vi "play sound rt.vi"() -> ()   [LabVIEW 2026]
uses:
  <vilib>/Analysis/1siggen.llb/Ramp Pattern by Samples.vi
  68eb3da8-f18c-44af-9a6e-03eb1aa6e4d3.vi
  <vilib>/DAQmx/write.llb/DAQmx Write (Analog Wfm 1Chan NSamp).vi
  <vilib>/DAQmx/create/channels.llb/DAQmx Create Channel (AO-Voltage-Basic).vi
  <vilib>/DAQmx/configure/timing.llb/DAQmx Timing (Sample Clock).vi
  <vilib>/DAQmx/miscellaneous.llb/DAQmx Fill In Error Info.vi
  <resource>/objmgr/daqmx.rc
  <vilib>/Analysis/NI_AALBase.lvlib
panel:
  out "error out":errorcluster
  in  "stop":bool
  in  "Boolean":bool
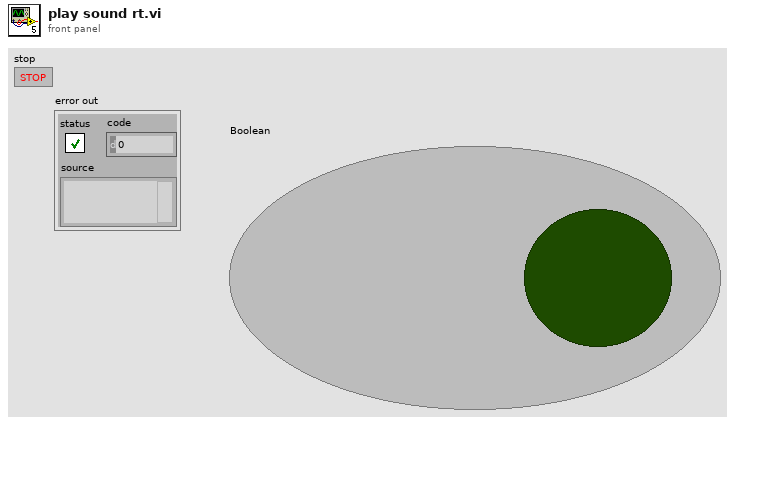
[diagram p1: front panel]
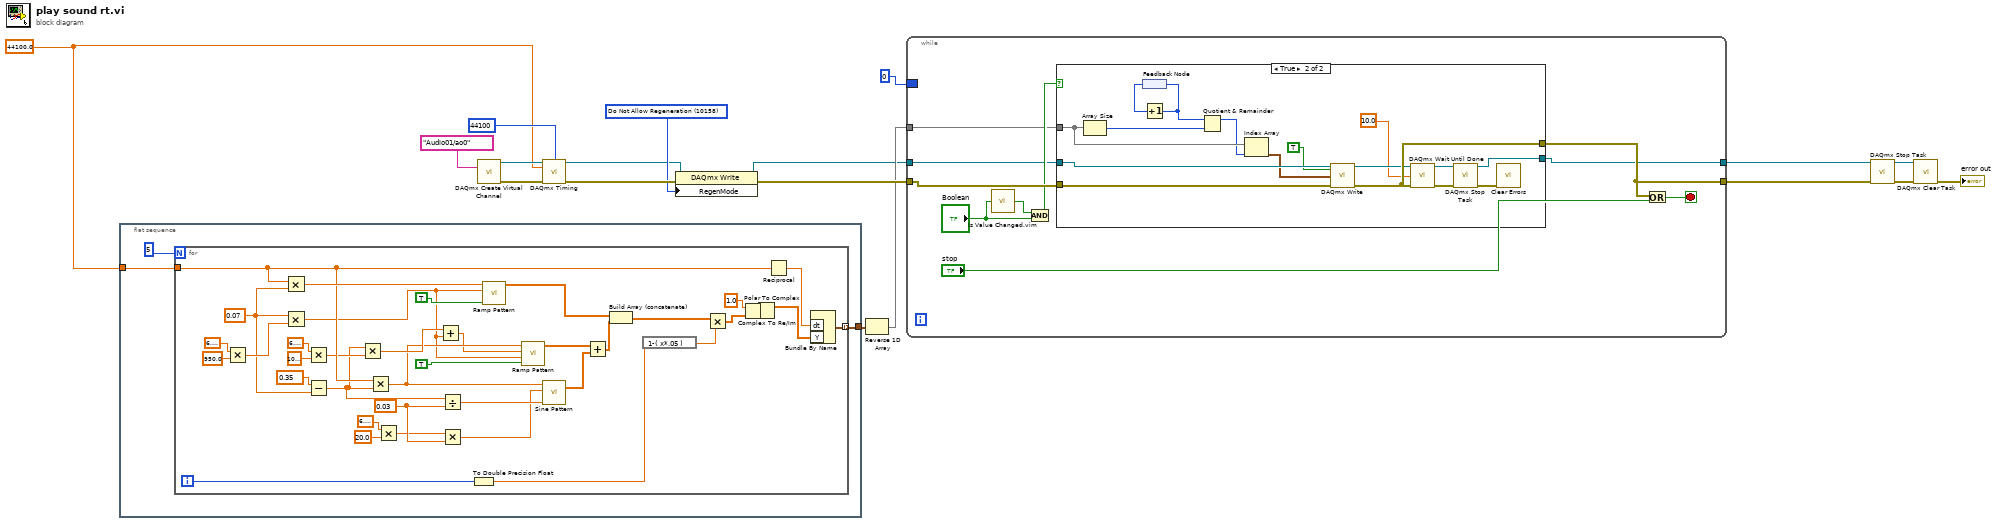
[diagram p0: block diagram]
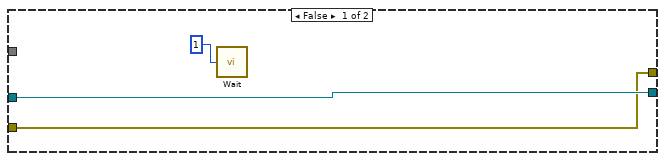
[diagram p2: hidden frame]
diagram:
  w7 = 10158 items=["Allow Regeneration"=10097, "Do Not Allow Regeneration"=10158] ("RegenMode")
  w5 = 44100.0 ("rate")
  n1 = flat-sequence {
    tunnel: [w21] -> w6
    tunnel: w5 -> [w20]
    frame #0 {
      n2 = for {
        N: 5 -> [_]
        tunnel: [w49] -> w21 mode=indexing
        tunnel: w20 -> [w45]
        i -> [w24]
        w33 = 0.03 ("y")
        w35 = 0.07 ("y")
        n3 = Multiply(x=6.283185307179586, y=950.0) -> (x*y=w55:dbl)
        n4 = Multiply(x=w45, y=w35) -> (x*y=w48:dbl)
        n5 = Multiply(x=w35, y=w55) -> (x*y=w26:dbl)
        n6 = Multiply(x=6.283185307179586, y=1000.0) -> (x*y=w41:dbl)
        n7 = Subtract(x=0.35 ("y"), y=w35) -> (x-y=w30:dbl)
        n8 = Multiply(x=w30, y=w41) -> (x*y=w47:dbl)
        n9 = Multiply(x=w45, y=w30) -> (x*y=w36:dbl)
        n10 = Multiply(x=6.283185307179586, y=20.0) -> (x*y=w32:dbl)
        n11 = Add(x=w47, y=w26) -> (x+y=w27:dbl)
        n12 = Divide(x=w30, y=w33) -> (x/y=w39:dbl)
        n13 = Multiply(x=w32, y=w33) -> (x*y=w31:dbl)
        n14 = To Double Precision Float(number=w24) -> (double precision float=w22:dbl)
        n15 = call-poly <vilib>:"Ramp Pattern.vi"("exclude end?"=TRUE, "end"=w26, "samples"=w48) -> ("Ramp Pattern"=w56:dbl[])  [unwired: 7 in, 1 out]
        n16 = call-poly <vilib>:"Ramp Pattern.vi"("exclude end?"=TRUE, "start"=w26, "end"=w27, "samples"=w36) -> ("Ramp Pattern"=w44:dbl[])  [unwired: 6 in, 1 out]
        n17 = call <vilib>:"Sine Pattern.vi"("cycles"=w39, "amplitude"=w31, "samples"=w36) -> ("Sinusoidal Pattern"=w34:dbl[])  [unwired: 1 in, 1 out]
        n18 = Add(x=w44, y=w34) -> (x+y=w28:dbl[])
        n19 = Build Array (concatenate)(w56, w28) -> (w29:dbl[])
        n20 = expression code="1-( x*.05 )"(w22) -> (w23:dbl)
        n21 = Multiply(x=w29, y=w23) -> (x*y=w25:dbl[])
        n22 = Polar To Complex(1:w25, 2:1.0 ("y")) -> (0:w52:cdb[])
        n23 = Complex To Re/Im(x + iy=w52) -> (x=w51:dbl[])  [unwired: 1 out]
        n24 = Reciprocal(x=w45) -> (1/x=w50:dbl)
        n25 = Bundle By Name("dt"=w50, "Y"=w51) -> (w49:waveform(dbl))  [unwired: 1 in]
      }
    }
  }
  n26 = call-poly <vilib>:"DAQmx Create Virtual Channel.vi"("physical channels"=tag "Audio01/ao0") -> ("task out"=w17:refnum<k21>, "error out"=w16:errorcluster)  [unwired: 13 in]
  n27 = call-poly <vilib>:"DAQmx Timing.vi"("task/channels in"=w17, "samples per channel"=44100, "rate"=w5, "error in"=w16) -> ("task out"=w2:refnum<k21>, "error out"=w15:errorcluster)  [unwired: 10 in]
  n28 = property class="DAQmx Write"(reference=w2, error in=w15, "RegenMode"=w7) -> (reference out=w1:refnum<k21>, error out=w8:errorcluster)
  n29 = Reverse 1D Array(array=w6) -> (reversed array=w4:waveform(dbl)[])
  n30 = while {
    tunnel: w1 -> [w62]
    tunnel: w8 -> [w68]
    tunnel: w4 -> [w59]
    tunnel: [w60] -> w13
    tunnel: [w61] -> w10
    border: u32 0 ("Count(Ticks)") -> [_]
    stop <- w66 stop-if-true
    n31 = call "Is Value Changed.vim"("value"="Boolean") -> ("changed or first call?"=w65:bool)
    n32 = And(x=w65, y="Boolean") -> (x .and. y?=w63:bool)
    n33 = case shown="True" w63 {
      tunnel: w62 -> [w71 w87]
      tunnel: w68 -> [w70 w86]
      tunnel: [w71 w80] -> w60
      tunnel: [w70 w85] -> w61
      tunnel: w59 -> [_ w76]
      frame False {
        n34 = call "Wait"("Count(Ticks)"=u32 1) -> ()  [unwired: 1 out]
      }
      frame True {
        n35 = Array Size(array=w76) -> (size(s)=w75:i32)
        n36 = feedback #1() -> (w73:u32)
        n37 = Increment(x=w73) -> (x+1=w74:u32)
        n38 = feedback-in #1(w74) -> ()
        n39 = Quotient & Remainder(x=w74, y=w75) -> (x-y*floor(x/y)=w72:u32)  [unwired: 1 out]
        n40 = Index Array(array=w76, index=w72) -> (element=w77:waveform(dbl))
        n41 = call-poly <vilib>:"DAQmx Write.vi"("task/channels in"=w87, "auto start"=TRUE, "data"=w77, "error in"=w86) -> ("task out"=w79:refnum<k21>, "error out"=w85:errorcluster)  [unwired: 9 in, 1 out]
        n42 = call <vilib>:"DAQmx Wait Until Done.vi"("task/channels in"=w79, "timeout (sec)"=10.0, "error in"=w85) -> ("task out"=w81:refnum<k21>, "error out"=w83:errorcluster)  [unwired: 11 in]
        n43 = call <vilib>:"DAQmx Stop Task.vi"("task/channels in"=w81, "error in"=w83) -> ("task out"=w80:refnum<k21>, "error out"=w82:errorcluster)  [unwired: 12 in]
        n44 = call <vilib>:"Clear Errors.vi"("error in (no error)"=w82) -> ()  [unwired: 5 in, 2 out]
      }
    }
    n45 = Or(x=w61, y="stop") -> (x .or. y?=w66:bool)
  }
  n46 = call <vilib>:"DAQmx Stop Task.vi"("task/channels in"=w13, "error in"=w10) -> ("task out"=w12:refnum<k21>, "error out"=w11:errorcluster)  [unwired: 12 in]
  n47 = call <vilib>:"DAQmx Clear Task.vi"("task in"=w12, "error in"=w11) -> ("error out"=→"error out":errorcluster)  [unwired: 13 in]
